vi "getSlitPosition.vi"(8 "error in (no error)":errorcluster, 10 "SlitType in":T2, 11 "Monochromator in":refnum<class "Monochromator.lvclass">) -> (0 "error out":errorcluster, 1 "Units":string, 2 "position":T1, 3 "Monochromator out":refnum<class "Monochromator.lvclass">)   [LabVIEW 2016, in "Monochromator.lvclass"]
uses:
  Monochromator.lvclass
  Typedefs/SlitType.ctl
  Typedefs/slitPosition.ctl
  Monochromator.lvclass/Monochromator.ctl
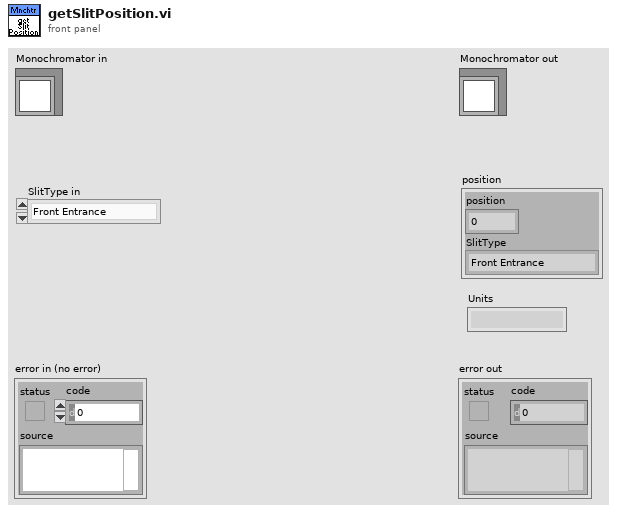
[diagram p1: front panel]
types:
  T1 = typedef "slitPosition.ctl" = cluster{"position":dbl, "SlitType":T2}
  T2 = typedef "SlitType.ctl" = enum16{"Front Entrance", "Side Entrance", "Front Exit", "Side Exit", "First Intermediate", "Second Intermediate"}
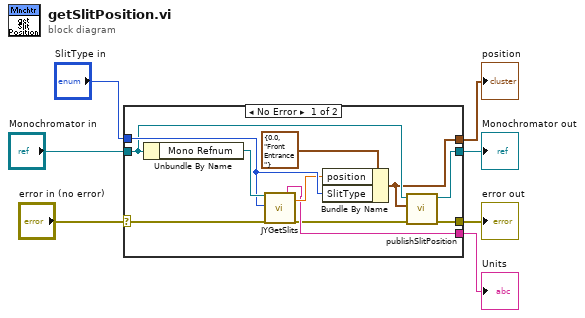
[diagram p0: block diagram]
diagram:
  n1 = case shown="No Error" "error in (no error)" {
    selector: "error in (no error)" -> [w17 w20]
    tunnel: [w11 w20] -> w6
    tunnel: [w9 w19] -> w4
    tunnel: "Monochromator in" -> [w10 w19]
    tunnel: "SlitType in" -> [w15 _]
    tunnel: [w8 _] -> w2
    tunnel: [w13 _] -> w1
    frame No Error {
      n2 = Unbundle By Name(w10) -> ("Mono Refnum"=w18:refnum<k7>)
      n3 = call "JYGetSlits.vi"("MonoRefNum IN"=w18, "Slit"=w15, "error in (no error)"=w17) -> ("Units"=w13:string, "Slit Width"=w14:dbl, "error out"=w12:errorcluster)  [unwired: 13 in, 1 out]
      n4 = Bundle By Name(cluster=T1 {"position"=0.0, "SlitType"=enum."Front Entrance"} ("position 2"), "position"=w14, "SlitType"=w15) -> (w8:T1)
      n5 = call "publishSlitPosition.vi"("error in (no error)"=w12, "slitPosition"=w8, "Monochromator in"=w10) -> ("error out"=w11:errorcluster, "Monochromator out"=w9:refnum<class "Monochromator.lvclass">)  [unwired: 7 in]
    }
    frame Error {
    }
  }
  "error out" <- w6
  "Monochromator out" <- w4
  "position" <- w2
  "Units" <- w1
